vi "Colonne da graficare.vi"(8 "Array 1ph":string[](array[string]), 9 "Array 3ph6ch":string[](array[string]), 10 "Array 3ph3ch":string[](array[string])) -> (0 "indici grafici m,3,6":T1[](array[typedef]), 1 "Array Array 1ph out":string[](array[string]), 2 "Array 3ph6ch out":string[](array[string]), 3 "Array 3ph3ch out":string[](array[string]))   [LabVIEW 2019]
uses:
  TypeDef/Indici.ctl
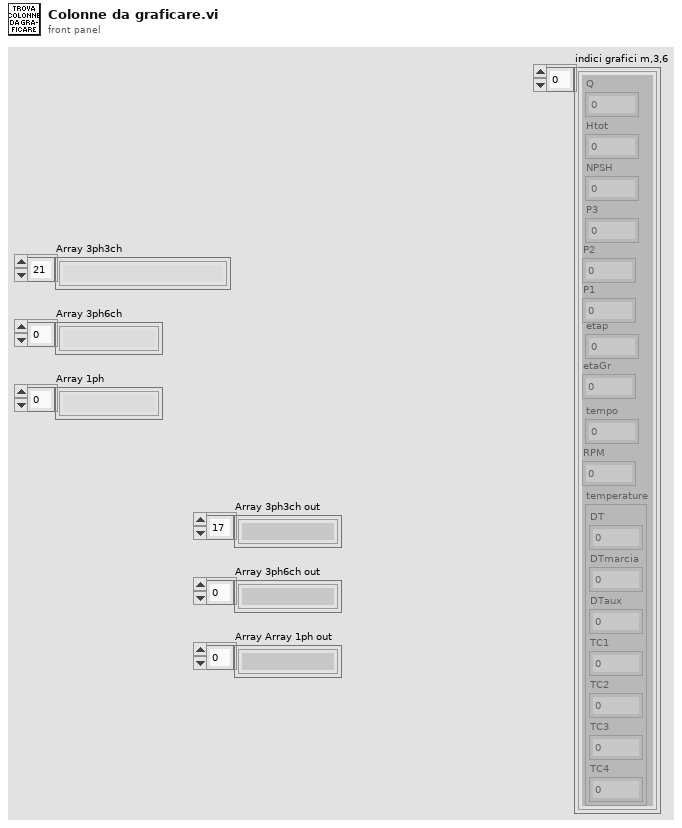
[diagram p1: front panel]
types:
  T1 = typedef "Indici.ctl" = cluster{"Q":i32, "Htot":i32, "NPSH":i32, "P3":i32, "etap":i32, "temperature":cluster{"DT":i32, "DTmarcia":i32, "DTaux":i32, "TC1":i32, "TC2":i32, "TC3":i32, "TC4":i32}, "tempo":i32, "P2":i32, "P1":i32, "etaGr":i32, "RPM":i32}
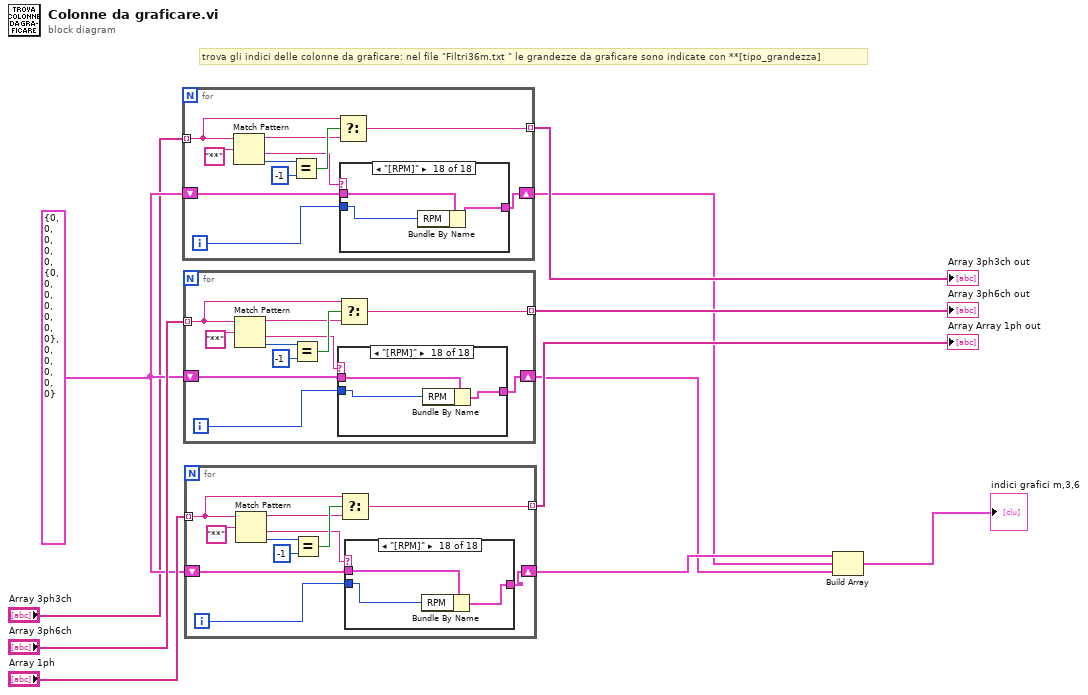
[diagram p0: block diagram]
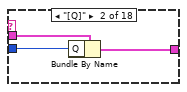
[diagram p3: hidden frame]
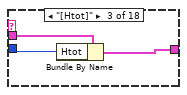
[diagram p4: hidden frame]
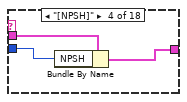
[diagram p5: hidden frame]
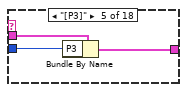
[diagram p6: hidden frame]
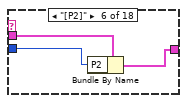
[diagram p7: hidden frame]
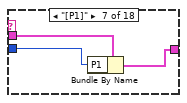
[diagram p8: hidden frame]
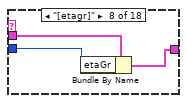
[diagram p9: hidden frame]
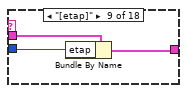
[diagram p10: hidden frame]
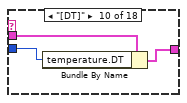
[diagram p11: hidden frame]
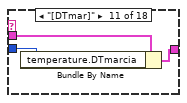
[diagram p12: hidden frame]
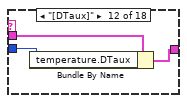
[diagram p13: hidden frame]
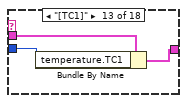
[diagram p14: hidden frame]
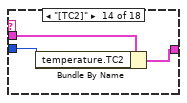
[diagram p15: hidden frame]
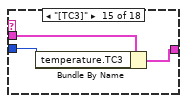
[diagram p16: hidden frame]
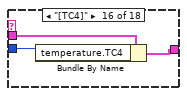
[diagram p17: hidden frame]
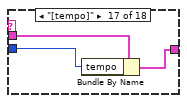
[diagram p18: hidden frame]
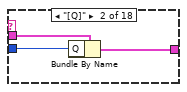
[diagram p20: hidden frame]
diagram:
  w2 = T1 {"Q"=0, "Htot"=0, "NPSH"=0, "P3"=0, "etap"=0, "temperature"={"DT"=0, "DTmarcia"=0, "DTaux"=0, "TC1"=0, "TC2"=0, "TC3"=0, "TC4"=0}, "tempo"=0, "P2"=0, "P1"=0, "etaGr"=0, "RPM"=0} ("indici")
  # "trova gli indici delle colonne da graficare: nel file \"Filtri36m.txt \" le grandezze da graficare sono indicate con **[tipo_grandezza]"
  n1 = for {
    tunnel: "Array 3ph3ch" -> [w16] mode=indexing
    tunnel: [w17] -> w6 mode=indexing
    shift-right: [w13] -> w5
    shift-left: w2 -> [w14]
    i -> [w12]
    n2 = Match Pattern(string=w16, regular expression="**") -> (before substring=w18:string, after substring=w15:string, offset past match=w21:i32)  [unwired: 1 in, 1 out]
    n3 = Equal?(x=w21, y=-1) -> (x = y?=w19:bool)
    n4 = Select(t=w16, s=w19, f=w18) -> (s? t:f=w17:string)
    n5 = case shown="\"[RPM]\"" w15 {
      tunnel: w14 -> [w23 w26 w29 w32 w35 w38 w41 w44 w47 w50 w53 w56 w59 w62 w65 w68 w71 w74]
      tunnel: [w23 w25 w27 w31 w33 w37 w40 w43 w45 w49 w52 w55 w58 w61 w64 w67 w70 w73] -> w13
      tunnel: w12 -> [_ w24 w28 w30 w34 w36 w39 w42 w46 w48 w51 w54 w57 w60 w63 w66 w69 w72]
      frame "False", Default {
      }
      frame "[Q]" {
        n6 = Bundle By Name(cluster=w26, "Q"=w24) -> (w25:T1)
      }
      frame "[Htot]" {
        n7 = Bundle By Name(cluster=w29, "Htot"=w28) -> (w27:T1)
      }
      frame "[NPSH]" {
        n8 = Bundle By Name(cluster=w32, "NPSH"=w30) -> (w31:T1)
      }
      frame "[P3]" {
        n9 = Bundle By Name(cluster=w35, "P3"=w34) -> (w33:T1)
      }
      frame "[P2]" {
        n10 = Bundle By Name(cluster=w38, "P2"=w36) -> (w37:T1)
      }
      frame "[P1]" {
        n11 = Bundle By Name(cluster=w41, "P1"=w39) -> (w40:T1)
      }
      frame "[etagr]" {
        n12 = Bundle By Name(cluster=w44, "etaGr"=w42) -> (w43:T1)
      }
      frame "[etap]" {
        n13 = Bundle By Name(cluster=w47, "etap"=w46) -> (w45:T1)
      }
      frame "[DT]" {
        n14 = Bundle By Name(cluster=w50, "temperature.DT"=w48) -> (w49:T1)
      }
      frame "[DTmar]" {
        n15 = Bundle By Name(cluster=w53, "temperature.DTmarcia"=w51) -> (w52:T1)
      }
      frame "[DTaux]" {
        n16 = Bundle By Name(cluster=w56, "temperature.DTaux"=w54) -> (w55:T1)
      }
      frame "[TC1]" {
        n17 = Bundle By Name(cluster=w59, "temperature.TC1"=w57) -> (w58:T1)
      }
      frame "[TC2]" {
        n18 = Bundle By Name(cluster=w62, "temperature.TC2"=w60) -> (w61:T1)
      }
      frame "[TC3]" {
        n19 = Bundle By Name(cluster=w65, "temperature.TC3"=w63) -> (w64:T1)
      }
      frame "[TC4]" {
        n20 = Bundle By Name(cluster=w68, "temperature.TC4"=w66) -> (w67:T1)
      }
      frame "[tempo]" {
        n21 = Bundle By Name(cluster=w71, "tempo"=w69) -> (w70:T1)
      }
      frame "[RPM]" {
        n22 = Bundle By Name(cluster=w74, "RPM"=w72) -> (w73:T1)
      }
    }
  }
  "Array 3ph3ch out" <- w6
  n23 = for {
    tunnel: "Array 3ph6ch" -> [w79] mode=indexing
    tunnel: [w80] -> w9 mode=indexing
    shift-right: [w78] -> w4
    shift-left: w2 -> [w77]
    i -> [w76]
    n24 = Match Pattern(string=w79, regular expression="**") -> (before substring=w81:string, after substring=w75:string, offset past match=w84:i32)  [unwired: 1 in, 1 out]
    n25 = Equal?(x=w84, y=-1) -> (x = y?=w82:bool)
    n26 = case shown="\"[RPM]\"" w75 {
      tunnel: w77 -> [w86 w89 w92 w95 w98 w101 w104 w107 w110 w113 w116 w119 w122 w125 w128 w131 w134 w137]
      tunnel: [w86 w88 w90 w94 w96 w100 w103 w106 w108 w112 w115 w118 w121 w124 w127 w130 w133 w136] -> w78
      tunnel: w76 -> [_ w87 w91 w93 w97 w99 w102 w105 w109 w111 w114 w117 w120 w123 w126 w129 w132 w135]
      frame "False", Default {
      }
      frame "[Q]" {
        n27 = Bundle By Name(cluster=w89, "Q"=w87) -> (w88:T1)
      }
      frame "[Htot]" {
        n28 = Bundle By Name(cluster=w92, "Htot"=w91) -> (w90:T1)
      }
      frame "[NPSH]" {
        n29 = Bundle By Name(cluster=w95, "NPSH"=w93) -> (w94:T1)
      }
      frame "[P3]" {
        n30 = Bundle By Name(cluster=w98, "P3"=w97) -> (w96:T1)
      }
      frame "[P2]" {
        n31 = Bundle By Name(cluster=w101, "P2"=w99) -> (w100:T1)
      }
      frame "[P1]" {
        n32 = Bundle By Name(cluster=w104, "P1"=w102) -> (w103:T1)
      }
      frame "[etagr]" {
        n33 = Bundle By Name(cluster=w107, "etaGr"=w105) -> (w106:T1)
      }
      frame "[etap]" {
        n34 = Bundle By Name(cluster=w110, "etap"=w109) -> (w108:T1)
      }
      frame "[DT]" {
        n35 = Bundle By Name(cluster=w113, "temperature.DT"=w111) -> (w112:T1)
      }
      frame "[DTmar]" {
        n36 = Bundle By Name(cluster=w116, "temperature.DTmarcia"=w114) -> (w115:T1)
      }
      frame "[DTaux]" {
        n37 = Bundle By Name(cluster=w119, "temperature.DTaux"=w117) -> (w118:T1)
      }
      frame "[TC1]" {
        n38 = Bundle By Name(cluster=w122, "temperature.TC1"=w120) -> (w121:T1)
      }
      frame "[TC2]" {
        n39 = Bundle By Name(cluster=w125, "temperature.TC2"=w123) -> (w124:T1)
      }
      frame "[TC3]" {
        n40 = Bundle By Name(cluster=w128, "temperature.TC3"=w126) -> (w127:T1)
      }
      frame "[TC4]" {
        n41 = Bundle By Name(cluster=w131, "temperature.TC4"=w129) -> (w130:T1)
      }
      frame "[tempo]" {
        n42 = Bundle By Name(cluster=w134, "tempo"=w132) -> (w133:T1)
      }
      frame "[RPM]" {
        n43 = Bundle By Name(cluster=w137, "RPM"=w135) -> (w136:T1)
      }
    }
    n44 = Select(t=w79, s=w82, f=w81) -> (s? t:f=w80:string)
  }
  "Array 3ph6ch out" <- w9
  n45 = for {
    tunnel: "Array 1ph" -> [w142] mode=indexing
    tunnel: [w143] -> w10 mode=indexing
    shift-right: [w139] -> w11
    shift-left: w2 -> [w141]
    i -> [w138]
    n46 = Match Pattern(string=w142, regular expression="**") -> (before substring=w144:string, after substring=w140:string, offset past match=w147:i32)  [unwired: 1 in, 1 out]
    n47 = Equal?(x=w147, y=-1) -> (x = y?=w145:bool)
    n48 = Select(t=w142, s=w145, f=w144) -> (s? t:f=w143:string)
    n49 = case shown="\"[RPM]\"" w140 {
      tunnel: w141 -> [w149 w152 w155 w158 w161 w164 w167 w170 w173 w176 w179 w182 w185 w188 w191 w194 w197 w200]
      tunnel: [w149 w151 w153 w157 w159 w163 w166 w169 w171 w175 w178 w181 w184 w187 w190 w193 w196 w199] -> w139
      tunnel: w138 -> [_ w150 w154 w156 w160 w162 w165 w168 w172 w174 w177 w180 w183 w186 w189 w192 w195 w198]
      frame "False", Default {
      }
      frame "[Q]" {
        n50 = Bundle By Name(cluster=w152, "Q"=w150) -> (w151:T1)
      }
      frame "[Htot]" {
        n51 = Bundle By Name(cluster=w155, "Htot"=w154) -> (w153:T1)
      }
      frame "[NPSH]" {
        n52 = Bundle By Name(cluster=w158, "NPSH"=w156) -> (w157:T1)
      }
      frame "[P3]" {
        n53 = Bundle By Name(cluster=w161, "P3"=w160) -> (w159:T1)
      }
      frame "[P2]" {
        n54 = Bundle By Name(cluster=w164, "P2"=w162) -> (w163:T1)
      }
      frame "[P1]" {
        n55 = Bundle By Name(cluster=w167, "P1"=w165) -> (w166:T1)
      }
      frame "[etagr]" {
        n56 = Bundle By Name(cluster=w170, "etaGr"=w168) -> (w169:T1)
      }
      frame "[etap]" {
        n57 = Bundle By Name(cluster=w173, "etap"=w172) -> (w171:T1)
      }
      frame "[DT]" {
        n58 = Bundle By Name(cluster=w176, "temperature.DT"=w174) -> (w175:T1)
      }
      frame "[DTmar]" {
        n59 = Bundle By Name(cluster=w179, "temperature.DTmarcia"=w177) -> (w178:T1)
      }
      frame "[DTaux]" {
        n60 = Bundle By Name(cluster=w182, "temperature.DTaux"=w180) -> (w181:T1)
      }
      frame "[TC1]" {
        n61 = Bundle By Name(cluster=w185, "temperature.TC1"=w183) -> (w184:T1)
      }
      frame "[TC2]" {
        n62 = Bundle By Name(cluster=w188, "temperature.TC2"=w186) -> (w187:T1)
      }
      frame "[TC3]" {
        n63 = Bundle By Name(cluster=w191, "temperature.TC3"=w189) -> (w190:T1)
      }
      frame "[TC4]" {
        n64 = Bundle By Name(cluster=w194, "temperature.TC4"=w192) -> (w193:T1)
      }
      frame "[tempo]" {
        n65 = Bundle By Name(cluster=w197, "tempo"=w195) -> (w196:T1)
      }
      frame "[RPM]" {
        n66 = Bundle By Name(cluster=w200, "RPM"=w198) -> (w199:T1)
      }
    }
  }
  "Array Array 1ph out" <- w10
  n67 = Build Array(w11, w5, w4) -> (→"indici grafici m,3,6":T1[])
